vi "AddLibSectionIfMissing.vi"(8 "error in (no error)":errorcluster, 10 "LibraryName":string="ModuleA", 11 "Config Refnum in":T1) -> (0 "error out":errorcluster, 3 "Config Refnum out":T1)   [LabVIEW 2019, in "Hawkeye.lvlib"]
uses:
  Hawkeye.lvlib
  <vilib>/Utility/config.llb/Config Data RefNum.ctl
  <vilib>/Utility/config.llb/Write Key (String).vi
  <vilib>/Utility/config.llb/NI_LVConfig.lvlib
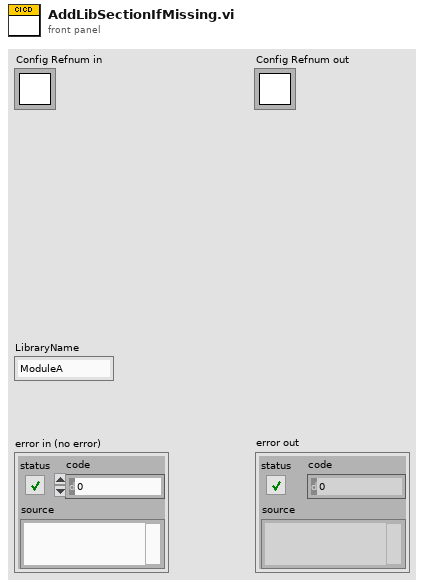
[diagram p1: front panel]
types:
  T1 = typedef "NI_LVConfig.lvlib/Config Data RefNum.ctl" = refnum<k1>
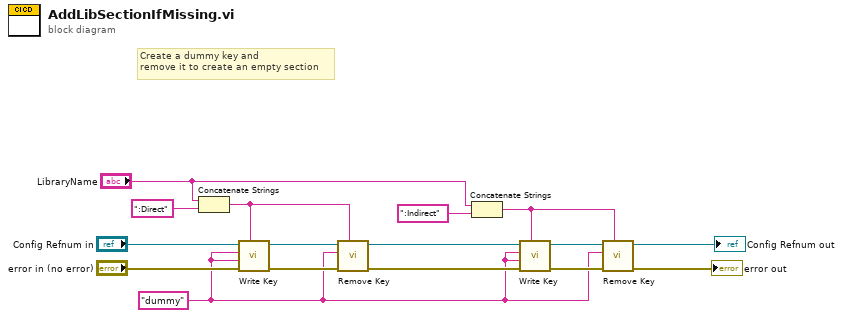
[diagram p0: block diagram]
diagram:
  w1 = "dummy" ("key")
  # "Create a dummy key and\nremove it to create an empty section"
  n1 = Concatenate Strings("LibraryName", ":Direct" ("Type")) -> (w2:string)
  n2 = call-poly <vilib>:"Write Key.vi"("section"=w2, "error in (no error)"="error in (no error)", "value"=w1, "key"=w1, "refnum"="Config Refnum in") -> ("error out"=w13:errorcluster, "refnum out"=w14:T1)  [unwired: 4 in, 1 out]
  n3 = call <vilib>:"Remove Key.vi"("section"=w2, "error in (no error)"=w13, "key"=w1, "refnum"=w14) -> ("error out"=w5:errorcluster, "refnum out"=w8:T1)  [unwired: 5 in, 1 out]
  n4 = Concatenate Strings("LibraryName", ":Indirect" ("Type")) -> (w4:string)
  n5 = call-poly <vilib>:"Write Key.vi"("section"=w4, "error in (no error)"=w5, "value"=w1, "key"=w1, "refnum"=w8) -> ("error out"=w10:errorcluster, "refnum out"=w9:T1)  [unwired: 4 in, 1 out]
  n6 = call <vilib>:"Remove Key.vi"("section"=w4, "error in (no error)"=w10, "key"=w1, "refnum"=w9) -> ("error out"=→"error out":errorcluster, "refnum out"=→"Config Refnum out":T1)  [unwired: 5 in, 1 out]
